vi "Initialize Async RT-RT.vi"(6 "Parameters":T9[](array[typedef]) {"Base Word" format="%04d"}, 8 "error in (no error)":errorcluster, 9 "Transmit Message Config":T8={"Tx Command Config"={"Command Type"=enum."Transmit", "Terminal Address"=enum."0", "SubAddress"=enum."1", "Word Count\\Mode Code"=enum."1", "Command Data"=[]}}, 10 "Receive Message Config":T1={"Group"=0, "High Priority"=FALSE, "Time to Next Msg (100 us)"=0, "Command Config"={"Command Type"=enum."Transmit", "Terminal Address"=enum."0", "SubAddress"=enum."1", "Word Count\\Mode Code"=enum."1", "Command Data"=[]}, "Message Control"={"MC17 Time Sync"=FALSE, "Error Mask"=FALSE, "Service Request Mask"=FALSE, "Busy Mask"=FALSE, "SubSystem Flag Mask"=FALSE, "Terminal Flag Mask"=FALSE, "Reserved Mask"=FALSE, "Retry"=FALSE, "Bus A / !Bus B"=FALSE, "Self-Test Loopback"=FALSE, "Broadcast Mask"=FALSE, "EoM Interrupt"=FALSE, "Mode Code Format"=FALSE, "Broadcast Format"=FALSE, "RT-RT Format"=FALSE}} {"Group" format="%04x"}, 11 "ID":string) -> (0 "error out":errorcluster, 3 "Async RT-RT Message out":refnum<class "Async RT-RT Message.lvclass">)   [LabVIEW 2020, in "BCI-1553 API.lvlib" / "Async RT-RT Message.lvclass"]
doc: "Generates an RT-to-RT Asynchronous Message object that can be sent out from a Bus Controller subcomponent after it has started. The RT-RT Async Message has all the same properties as an Asynchronous Message. An RT-RT Async Message can be high or low priority. High priority Messages get sent out as soon as there is time to do so in-between the execution of Messages. Low priority Messages are sent out between the execution of Minor Frames, if there is enough time to do so. The Group value should always be set to 0.\n\nThe Async Message Config contains the definition for the receive command. The RT-RT Async Message Config contains the definition for the transmit command."
uses:
  Async RT-RT Message.lvclass
  TypeDefs/Simplified Parameter Data Table.ctl
  TypeDefs/Scaling Information.ctl
  TypeDefs/Async RT-RT Message Config.ctl
  TypeDefs/Command Config.ctl
  TypeDefs/Command Type.ctl
  TypeDefs/Command Terminal Address.ctl
  TypeDefs/Command SubAddress.ctl
  TypeDefs/Command Word Count.ctl
  TypeDefs/Async Message Config.ctl
  TypeDefs/Message Control.ctl
  TypeDefs/Parameter Table Data.ctl
  Async RT-RT Message.lvclass/Async RT-RT Message.ctl
  BCI-1553 API.lvlib
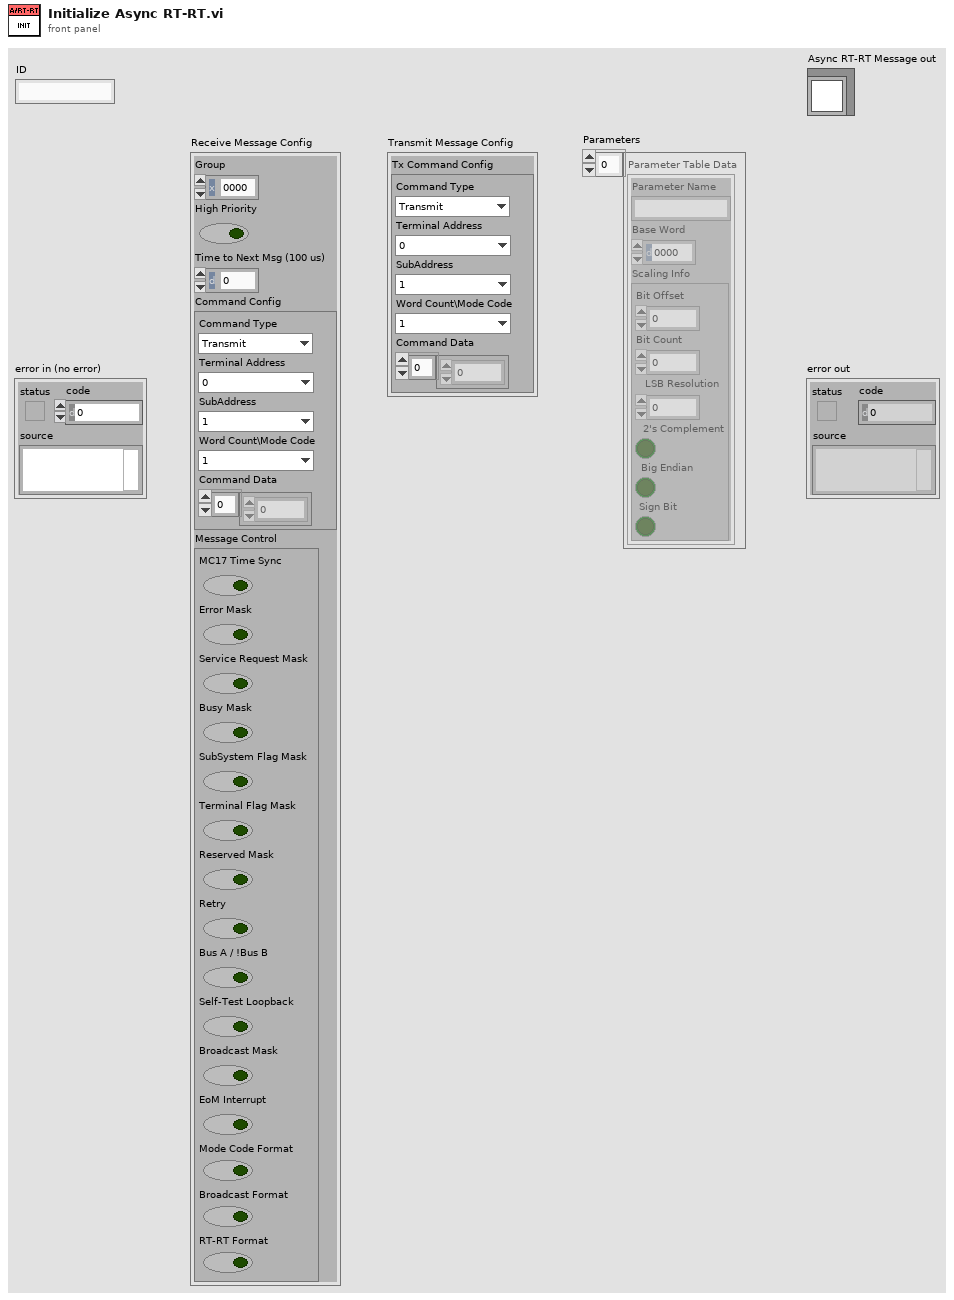
[diagram p1: front panel]
types:
  T1 = typedef "BCI-1553 API.lvlib/Async Message Config.ctl" = cluster{"Group":i32, "High Priority":bool, "Time to Next Msg (100 us)":u16, "Command Config":T2, "Message Control":T7}
  T2 = typedef "BCI-1553 API.lvlib/Command Config.ctl" = cluster{"Command Type":T3, "Terminal Address":T4, "SubAddress":T5, "Word Count\\Mode Code":T6, "Command Data":u16[]}
  T3 = typedef "BCI-1553 API.lvlib/Command Type.ctl" = enum16{"Transmit", "Receive"}
  T4 = typedef "BCI-1553 API.lvlib/Command Terminal Address.ctl" = enum16{"0", "1", "2", "3", "4", "5", "6", "7", "8", "9", "10", "11", "12", "13", "14", "15", "16", "17", "18", "19", "20", "21", "22", "23", "24", "25", "26", "27", "28", "29", "30", "Broadcast"}
  T5 = typedef "BCI-1553 API.lvlib/Command SubAddress.ctl" = enum16{"Mode Code", "1", "2", "3", "4", "5", "6", "7", "8", "9", "10", "11", "12", "13", "14", "15", "16", "17", "18", "19", "20", "21", "22", "23", "24", "25", "26", "27", "28", "29", "30"}
  T6 = typedef "BCI-1553 API.lvlib/Command Word Count.ctl" = enum16{"1", "2", "3", "4", "5", "6", "7", "8", "9", "10", "11", "12", "13", "14", "15", "16", "17", "18", "19", "20", "21", "22", "23", "24", "25", "26", "27", "28", "29", "30", "31", "32"}
  T7 = typedef "BCI-1553 API.lvlib/Message Control.ctl" = cluster{"MC17 Time Sync":bool, "Error Mask":bool, "Service Request Mask":bool, "Busy Mask":bool, "SubSystem Flag Mask":bool, "Terminal Flag Mask":bool, "Reserved Mask":bool, "Retry":bool, "Bus A / !Bus B":bool, "Self-Test Loopback":bool, "Broadcast Mask":bool, "EoM Interrupt":bool, "Mode Code Format":bool, "Broadcast Format":bool, "RT-RT Format":bool}
  T8 = typedef "BCI-1553 API.lvlib/Async RT-RT Message Config.ctl" = cluster{"Tx Command Config":T2}
  T9 = typedef "BCI-1553 API.lvlib/Simplified Parameter Data Table.ctl" = cluster{"Parameter Name":string, "Base Word":u16, "Scaling Info":T10}
  T10 = typedef "BCI-1553 API.lvlib/Scaling Information.ctl" = cluster{"Bit Offset":i32, "Bit Count":i32, "LSB Resolution":dbl, "2's Complement":bool, "Big Endian":bool, "Sign Bit":bool}
  T11 = typedef "BCI-1553 API.lvlib/Parameter Table Data.ctl" = cluster{"Parameter Name":string, "Base Word":u16, "Address":u16, "Value":u64, "Mask":u16[], "Scaling Info":T10}
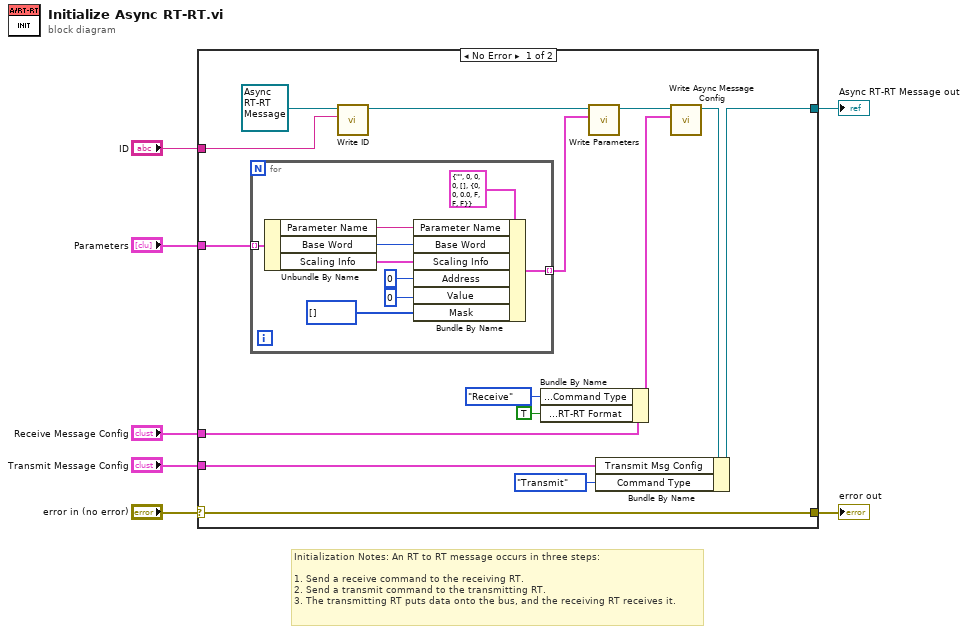
[diagram p0: block diagram]
diagram:
  # "Initialization Notes: An RT to RT message occurs in three steps:\n\n1. Send a receive command to the receiving RT.\n2. Send a transmit command to the transmitting RT.\n3. The transmitting RT puts data onto the bus, and the receiving RT receives it."
  n1 = case shown="No Error" "error in (no error)" {
    selector: "error in (no error)" -> [w22 w32]
    tunnel: [w22 w32] -> w6
    tunnel: [w17 _] -> w5
    tunnel: "ID" -> [w20 _]
    tunnel: "Parameters" -> [w14 _]
    tunnel: "Transmit Message Config" -> [w18 _]
    tunnel: "Receive Message Config" -> [w12 _]
    frame No Error {
      n2 = for {
        tunnel: w14 -> [w29] mode=indexing
        tunnel: [w30] -> w13 mode=indexing
        n3 = Unbundle By Name(w29) -> ("Parameter Name"=w28:string, "Base Word"=w27:u16, "Scaling Info"=w23:T10)
        n4 = Bundle By Name(cluster=T11 {"Parameter Name"="", "Base Word"=0, "Address"=0, "Value"=0, "Mask"=[], "Scaling Info"={"Bit Offset"=0, "Bit Count"=0, "LSB Resolution"=0.0, "2's Complement"=FALSE, "Big Endian"=FALSE, "Sign Bit"=FALSE}} ("Parameter Table Data"), "Parameter Name"=w28, "Base Word"=w27, "Scaling Info"=w23, "Address"=u16 0, "Value"=u64 0, "Mask"=u16[] []) -> (w30:T11)
      }
      n5 = call-dynamic "Write ID.vi"("ID"=w20, "Async Message in"=refnum<class "Async RT-RT Message.lvclass"> refnum ("Async RT-RT Message out")) -> ("Async Message out"=w19:refnum<class "Async RT-RT Message.lvclass">)  [unwired: 8 in, 1 out]
      n6 = Bundle By Name(cluster=w12, "Command Config.Command Type"=Command_Type."Receive", "Message Control.RT-RT Format"=TRUE) -> (w11:T1)
      n7 = call-dynamic "Write Parameters.vi"("Parameters"=w13, "Async Message in"=w19) -> ("Async Message out"=w16:refnum<class "Async RT-RT Message.lvclass">)  [unwired: 8 in, 1 out]
      n8 = call-dynamic "Write Async Message Config.vi"("Async Message Config"=w11, "Async Message in"=w16) -> ("Async Message out"=w15:refnum<class "Async RT-RT Message.lvclass">)  [unwired: 8 in, 1 out]
      n9 = Bundle By Name(cluster=w15, "Transmit Msg Config"=w18, "Command Type"=Command_Type."Transmit" ("Transmit Msg Config.Tx Command Config.Command Type")) -> (w17:refnum<class "Async RT-RT Message.lvclass">)
    }
    frame Error {
    }
  }
  "error out" <- w6
  "Async RT-RT Message out" <- w5
